vi "Main_PXI_v2.0.vi"() -> ()   [LabVIEW 2018]
doc: "Main VI for the controls"
uses:
  components/pmcl dynamic signal analyzer/Controls/DSA excitation specs.ctl
  components/pmcl dynamic signal analyzer/Controls/DSA cycle specs.ctl
  Typedefs/StateDef_Enum.ctl
  <vilib>/Utility/error.llb/DialogType.ctl
  <vilib>/Platform/TimedLoop/XDataNode/timing_clust.ctl
  <vilib>/Platform/TimedLoop/XDataNode/nitl_modes.ctl
  <vilib>/Platform/TimedLoop/XDataNode/wakeup.ctl
  <vilib>/DAQmx/read.llb/DAQmx Read (Analog 1D DBL NChan 1Samp).vi
  <vilib>/DAQmx/write.llb/DAQmx Write (Analog DBL 1Chan 1Samp).vi
  <vilib>/DAQmx/create/channels.llb/DAQmx Create Channel (AO-Voltage-Basic).vi
  <vilib>/DAQmx/create/channels.llb/DAQmx Create Channel (AI-Voltage-Basic).vi
  <vilib>/DAQmx/configure/timing.llb/DAQmx Timing (Sample Clock).vi
  <vilib>/DAQmx/create/timing.llb/DAQmx Create Timing Source (Control Loop From Task).vi
  <vilib>/DAQmx/miscellaneous.llb/DAQmx Fill In Error Info.vi
  <vilib>/Platform/TimedLoop/XDataNode/XDataNode.xnode
  Components/Timing/Timing.lvlib
  <vilib>/Platform/TimedLoop/XDataNode/XDNodeRunTimeDep.lvlib
  <vilib>/Analysis/NI_AALPro.lvlib
  <vilib>/ptbypt/NI_PtbyPt.lvlib
  <resource>/objmgr/daqmx.rc
  Components/Controller/Controller.lvlib
panel:
  in  "System Stop Button":bool
  in  "Pause chart?":bool
  in  "Controller Params":enum32{"Page 1"}(tab)
  in  "Kp":dbl=1.0 min=0.0
  in  "Controller On?":bool
  out "Status":string
  in  "Ref. Gen.":enum32{"Analog In", "Manual", "Wave Gen", "DSA"}(tab)=enum."Manual"
  in  "Ref. cmd.":dbl(slide) step=1.0 scale=-10.0..10.0 scale format="%#.1f"
  in  "Signal Cluster":T1={"phase"=0.0, "amplitude"=1.0, "frequency"=1.0, "offset"=1.0, "Signal"=enum."Square"} {"offset" format="%0.2f"; "frequency" format="%0.2f"; "amplitude" format="%0.2f"; "phase" format="%0.2f"}
  in  "Frequency\nResponse":enum16{"Plant", "RR", "CL"}(ring)
  out "DSA \nRunning?":bool
  in  "Stop \nDSA":bool
  in  "Start \nDSA":bool
  in  "DSA excitation specs":T2={"Initial Freq. [Hz]"=10.0, "Final Freq. [Hz]"=999.0, "# pts. in interval"=50, "Samping Time [s]"=0.001, "Amplitude [V]"=1.0, "Offset [V]"=0.0, "Freq Units (F: rad/s, T: Hz)"=TRUE}
  in  "Cycle Specs":T3={"Cycles To \nSettle (M)"=5, "Cycles To \nCalculate (N)"=10}
  in  "Loop Timing":enum32{"Ctrl.", "Ref. gen", "UI"}(tab)
  in  "ConvLateErrToWarning?":bool=TRUE
  in  "Ctrl.\nLoop Rate (Hz)":dbl=25000.0 format="%#_4p"
  out "# Finished\nLate counter":dbl
  out "# Finished\nLate counter":dbl
  in  "Ref. Gen.\nLoop Rate (Hz)":dbl=20000.0 format="%#_4p"
  in  "UI Loop rate (Hz)":dbl=1000.0 format="%#_6p"
  in  "Display Waveforms":enum32{"Controller Signals", "DSA "}(tab)
  out "Control Effort":dbl(graph)
  out "Waveform Chart":cluster{"Double":dbl, "Numeric":dbl}(graph)
  out "Phase Bode Plot":cluster{dbl[], dbl[]}(graph)
  out "Magnitude Bode Plot":cluster{dbl[], dbl[]}(graph)
  out "DSA Signals":cluster{"Double":dbl, "Double":dbl}(graph)
  # "Connect the Reference Signal \nto C/AI 1 of the myRIO."
  # "Pinout Config.:\nPort C/AI0 : Plant output being read           by the controller.\nPort C/AI1 : Reference signal for the control loop.\nPort C/AO0 : Control effort signal to the plant."
  # "Control Loop Timing"
  # "Ref.  Gen. Loop Timing"
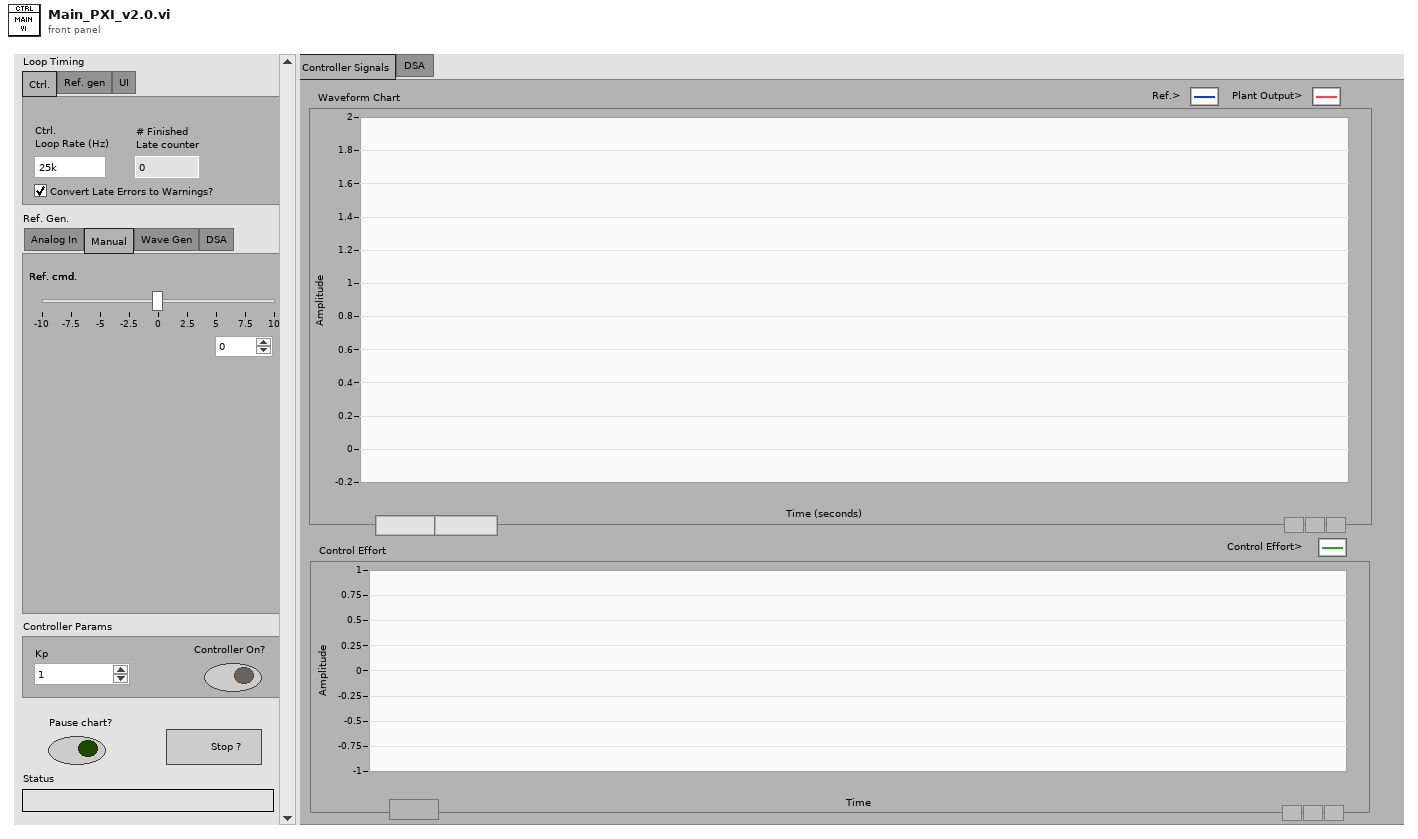
[diagram p1: front panel]
types:
  T1 = cluster{"phase":dbl, "amplitude":dbl, "frequency":dbl, "offset":dbl, "Signal":enum16{"Sine", "Square", "Sawtooth"}}
  T2 = typedef "DSA excitation specs.ctl" = cluster{"Initial Freq. [Hz]":dbl, "Final Freq. [Hz]":dbl, "# pts. in interval":i16, "Samping Time [s]":dbl, "Amplitude [V]":dbl, "Offset [V]":dbl, "Freq Units (F: rad/s, T: Hz)":bool}
  T3 = typedef "DSA cycle specs.ctl" = cluster{"Cycles To \nSettle (M)":i16, "Cycles To \nCalculate (N)":i16}
  T4 = typedef "DialogType.ctl" = u16
  T5 = typedef "StateDef_Enum.ctl" = enum16{"Initialize", "Wait", "Shutdown"}
  T6 = typedef "XDNodeRunTimeDep.lvlib/timing_clust.ctl" = cluster{"Expected End [f-1]":u64, "Actual End [f-1]":u64, "Finished Late? [f-1]":bool, "Expected End [i-1]":u64, "Actual End [i-1]":u64, "Finished Late? [i-1]":bool, "Expected Start [i]":u64, "Actual Start [i]":u64, "Expected Start [f]":u64, "Actual Start [f]":u64, "Source Name":string, "Structure Name":string, "Period":i64, "Deadline":i64, "Offset":i64, "Start":i64, "Priority":i32, "Timeout":i32, "Mode":T7, "Wakeup Reason":T8, "Error":errorcluster, "Source Type":string, "Secondary Source Type":string, "Global End Time":u64, "Global Start Time":u64, "Frame Duration":u64, "Iteration Duration":u64, "Assigned CPU":i32, "I/O Scan Engine Mode":u32}
  T7 = typedef "XDNodeRunTimeDep.lvlib/nitl_modes.ctl" = enum32{"No Change", "Process missed periods, maintain original phase", "Discard missed periods, maintain original phase", "Process missed periods, ignore original phase", "Discard missed periods, ignore original phase"}
  T8 = typedef "XDNodeRunTimeDep.lvlib/wakeup.ctl" = enum32{"Normal", "Aborted", "Asynchronous wakeup", "Timing source error", "Timed loop error", "Timeout"}
  T9 = cluster{"Analog In CH1":dbl, "Analog In CH0":dbl}
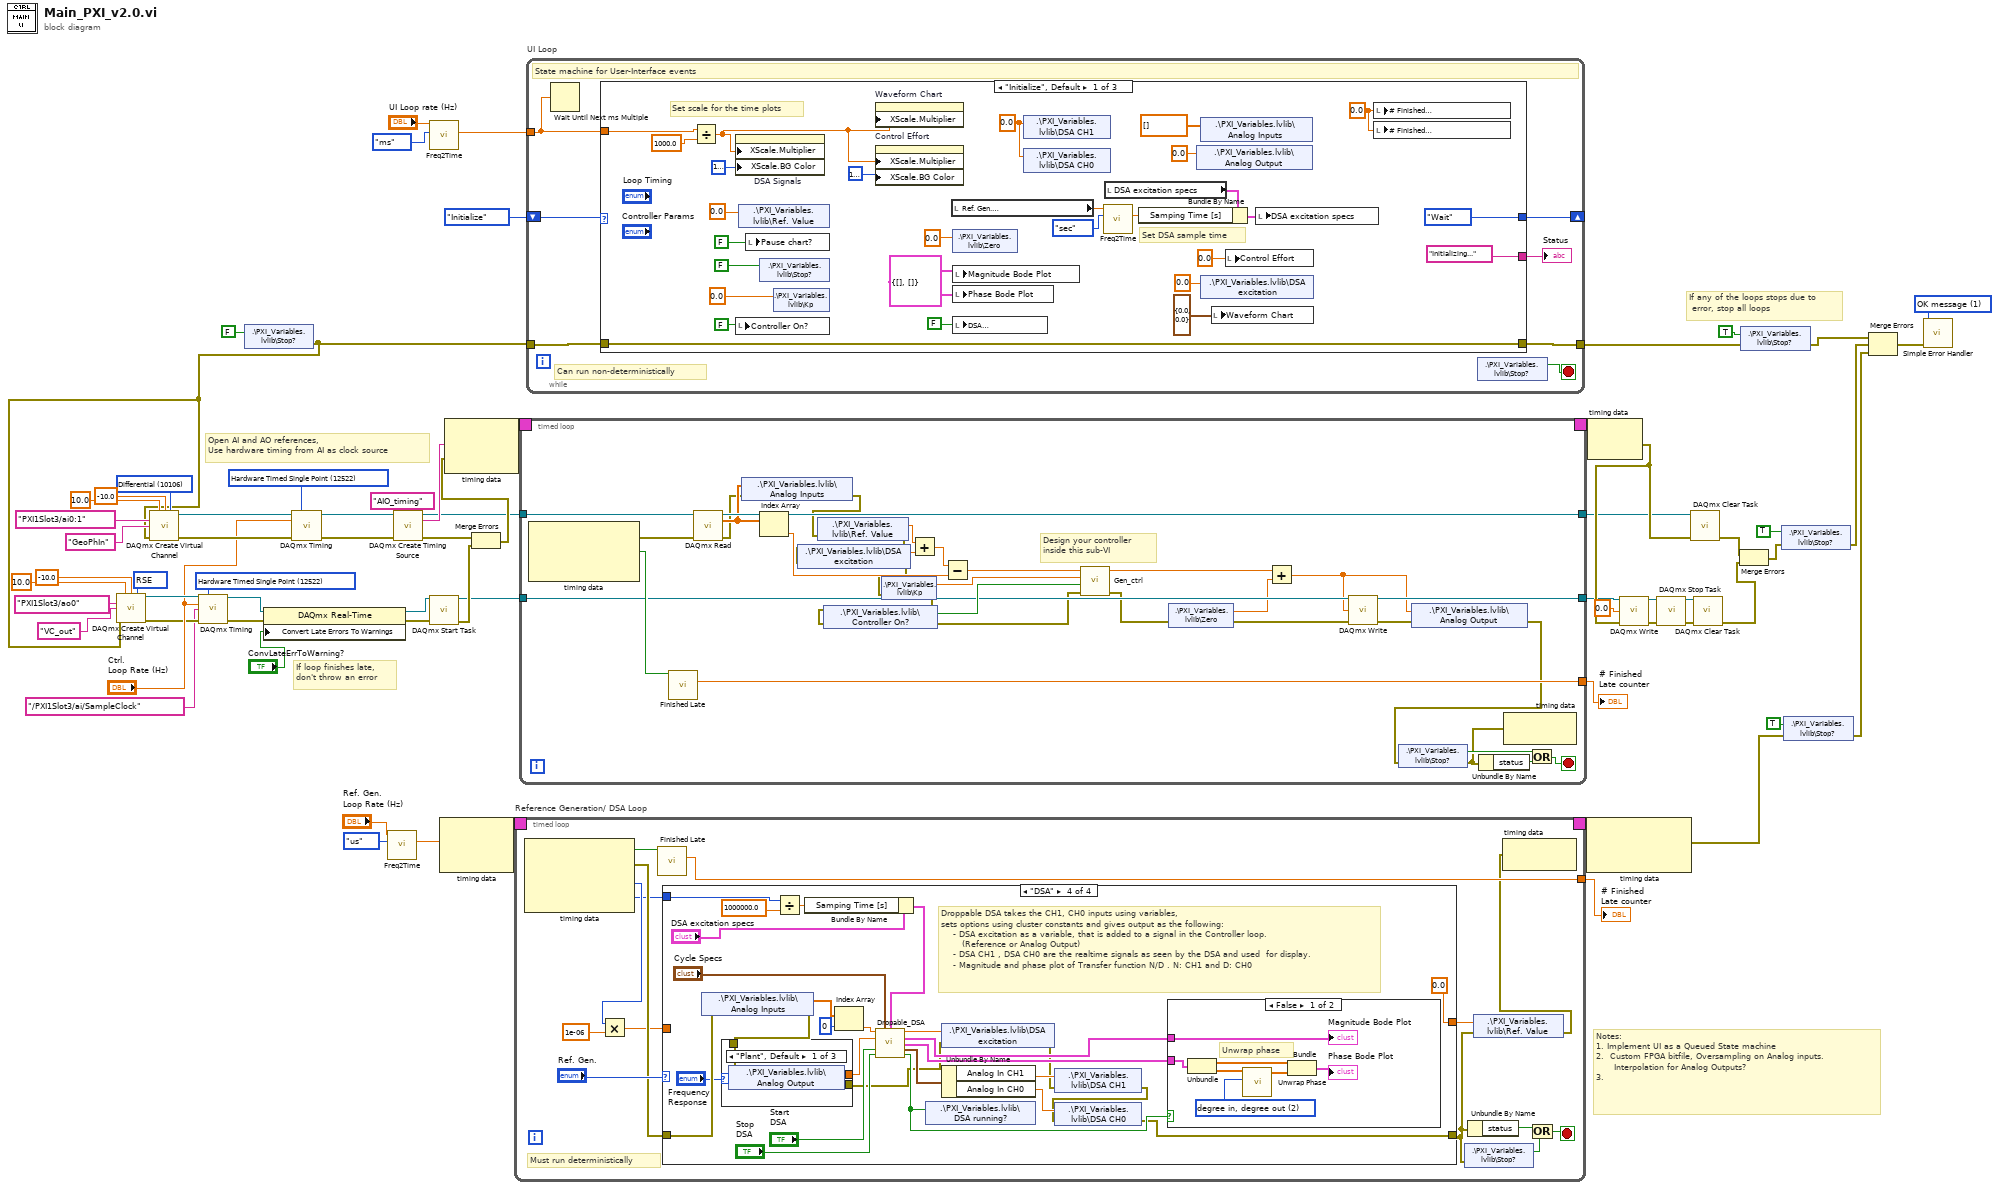
[diagram p0: block diagram]
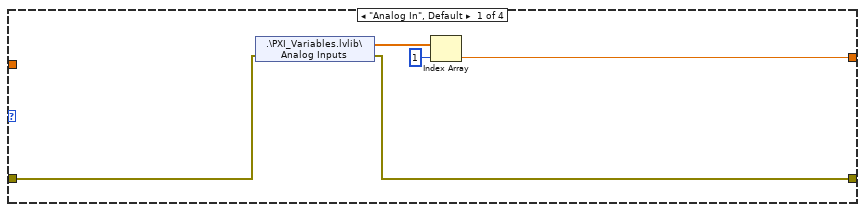
[diagram p2: hidden frame]
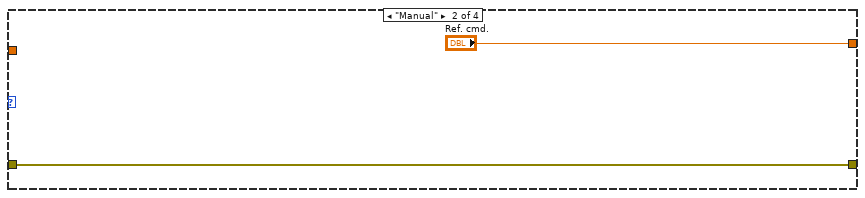
[diagram p3: hidden frame]
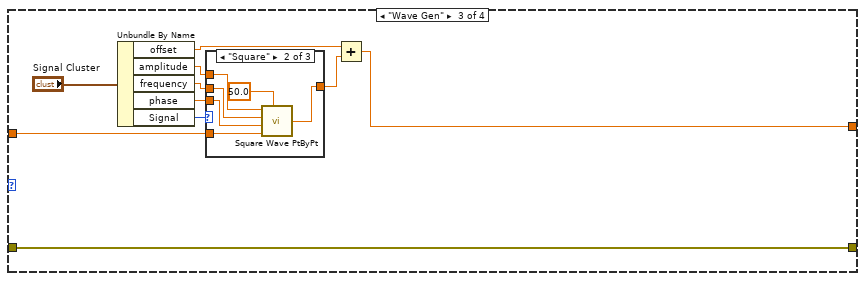
[diagram p4: hidden frame]
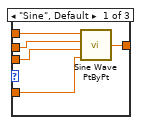
[diagram p5: hidden frame]
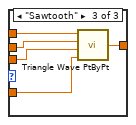
[diagram p6: hidden frame]
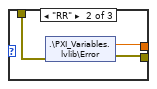
[diagram p7: hidden frame]
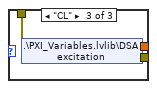
[diagram p8: hidden frame]
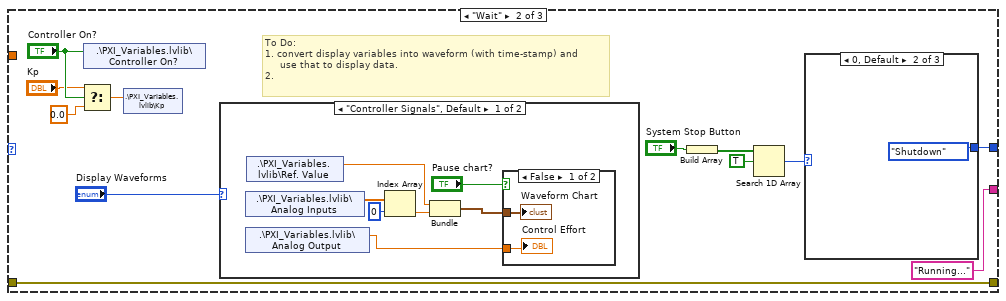
[diagram p10: hidden frame]
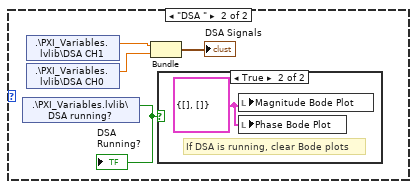
[diagram p12: hidden frame]
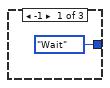
[diagram p14: hidden frame]
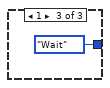
[diagram p15: hidden frame]
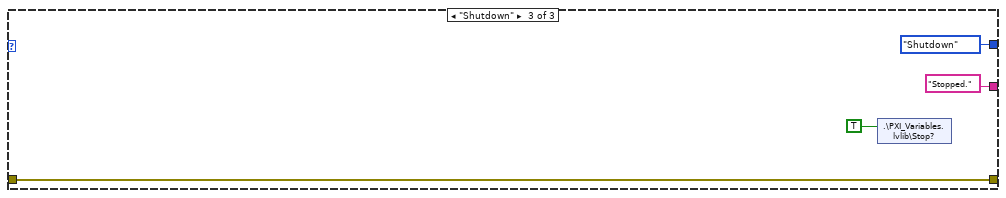
[diagram p16: hidden frame]
diagram:
  w7 = 12522 items=["Finite Samples"=10178, "Continuous Samples"=10123, "Hardware Timed Single Point"=12522] ("sample mode")
  w13 = T4 1 items=["no dialog", "OK message", "continue or stop message", "OK message + warnings", "continue/stop + warnings"] ("type of dialog (OK msg:1)")
  w22 = 12522 items=["Finite Samples"=10178, "Continuous Samples"=10123, "Hardware Timed Single Point"=12522] ("sample mode")
  w47 = 10106 items=["Default"=-1, "RSE"=10083, "NRSE"=10078, "Differential"=10106, "Pseudodifferential"=12529] ("input terminal configuration")
  w51 = 10083 items=["Default"=-1, "RSE"=10083, "Differential"=10106, "Pseudodifferential"=12529] ("output terminal configuration")
  # "If loop finishes late,\ndon't throw an error"
  # "Open AI and AO references,\nUse hardware timing from AI as clock source"
  # "Notes:\n1. Implement UI as a Queued State machine\n2.  Custom FPGA bitfile, Oversampling on Analog inputs. \n      Interpolation for Analog Outputs?\n3."
  # "If any of the loops stops due to\n error, stop all loops"
  n1 = shared-variable ".\\PXI_Variables.lvlib\\Stop?"(FALSE ("Stop?")) -> (error out=w4:errorcluster)  [unwired: 1 in]
  n2 = call-poly <vilib>:"DAQmx Create Virtual Channel.vi"("maximum value"=10.0, "minimum value"=-10.0, "output terminal configuration"=w51, "physical channels"=tag "PXI1Slot3/ao0", "name to assign"="VC_out", "error in"=w4) -> ("task out"=w12:refnum<k21>, "error out"=w8:errorcluster)  [unwired: 8 in]
  n3 = call-poly <vilib>:"DAQmx Create Virtual Channel.vi"("maximum value"=10.0, "minimum value"=-10.0, "input terminal configuration"=w47, "physical channels"=tag "PXI1Slot3/ai0:1", "name to assign"="GeoPhIn", "error in"=w4) -> ("task out"=w24:refnum<k21>, "error out"=w23:errorcluster)  [unwired: 8 in]
  n4 = call-poly <vilib>:"DAQmx Timing.vi"("task/channels in"=w12, "sample mode"=w7, "rate"="Ctrl.\nLoop Rate (Hz)", "source"=tag "/PXI1Slot3/ai/SampleClock", "error in"=w8) -> ("task out"=w10:refnum<k21>, "error out"=w9:errorcluster)  [unwired: 9 in]
  n5 = property class="DAQmx Real-Time"(reference=w10, error in=w9, "Convert Late Errors To Warnings"="ConvLateErrToWarning?") -> (reference out=w15:refnum<k21>, error out=w20:errorcluster)
  n6 = call-poly <vilib>:"DAQmx Timing.vi"("task/channels in"=w24, "sample mode"=w22, "rate"="Ctrl.\nLoop Rate (Hz)", "error in"=w23) -> ("task out"=w14:refnum<k21>, "error out"=w17:errorcluster)  [unwired: 10 in]
  n7 = call "Freq2Time.vi"("Int. Time Unit"=enum16{"sec", "us", "ms"}."us", "Sample rate (Hz)"="Ref. Gen.\nLoop Rate (Hz)") -> ("Int.  time [unit]"=w3:dbl)  [unwired: 7 in, 2 out]
  n8 = call-poly <vilib>:"DAQmx Create Timing Source.vi"("task/channels in"=w14, "timing source name"="AIO_timing", "error in"=w17) -> ("task out"=w18:refnum<k21>, "timing source out"=w19:string, "error out"=w16:errorcluster)  [unwired: 10 in]
  n9 = call "Freq2Time.vi"("Int. Time Unit"=enum16{"sec", "us", "ms"}."ms", "Sample rate (Hz)"="UI Loop rate (Hz)") -> ("Int.  time [unit]"=w59:dbl)  [unwired: 7 in, 2 out]
  n10 = call <vilib>:"DAQmx Start Task.vi"("task/channels in"=w15, "error in"=w20) -> ("task out"=w26:refnum<k21>, "error out"=w49:errorcluster)  [unwired: 12 in]
  n11 = node-c288(w3) -> (w66:T6)  [unwired: 1 in]
  n12 = Merge Errors(w16, w49) -> (w41:errorcluster)
  n13 = node-c288(w19, w41) -> (w43:T6)
  n14 = timed-loop "Reference Generation/ DSA Loop" {
    timing: w66 -> [_]
    timing-out: [_] -> w65
    tunnel: [w81] -> w64
    stop <- w75 stop-if-true
    # "Must run deterministically"
    n15 = node-c288() -> (w82:bool, w78:errorcluster, w72:i64, w71:i64)  [unwired: 1 in]
    n16 = Multiply(x=w72, y=1e-06) -> (x*y=w74:dbl)
    n17 = call "Finished Late.vi"("Finished \nLate?"=w82) -> ("# Finished\nLate counter"=w81:dbl)  [unwired: 8 in, 2 out]
    n18 = case shown="\"DSA\"" "Ref. Gen." {
      tunnel: [w87 "Ref. cmd." w92 0.0 ("Ref. cmd.")] -> w79
      tunnel: w78 -> [w85 w88 w91 w122]
      tunnel: [w84 w88 w91 w125] -> w69
      tunnel: w74 -> [_ _ w90 _]
      tunnel: w71 -> [_ _ _ w132]
      frame "Analog In", Default {
        n19 = shared-variable ".\\PXI_Variables.lvlib\\Analog Inputs"(error in=w85) -> (w86:dbl[], error out=w84:errorcluster)
        n20 = Index Array(array=w86, index=1) -> (element=w87:dbl)
      }
      frame "Manual" {
      }
      frame "Wave Gen" {
        n21 = Unbundle By Name("Signal Cluster") -> ("offset"=w93:dbl, "amplitude"=w96:dbl, "frequency"=w95:dbl, "phase"=w94:dbl, "Signal"=w97:enum16{"Sine", "Square", "Sawtooth"})
        n22 = case shown="\"Square\"" w97 {
          tunnel: [w104 w109 w115] -> w99
          tunnel: w96 -> [w103 w108 w114]
          tunnel: w95 -> [w102 w107 w113]
          tunnel: w94 -> [w101 w106 w112]
          tunnel: w90 -> [w100 w105 w111]
          frame "Sine", Default {
            n23 = call <vilib>:"Sine Wave PtByPt.vi"("time"=w100, "phase"=w101, "frequency"=w102, "amplitude"=w103) -> ("sine wave"=w104:dbl)
          }
          frame "Square" {
            n24 = call <vilib>:"Square Wave PtByPt.vi"("amplitude"=w108, "frequency"=w107, "phase"=w106, "time"=w105, "duty cycle (%)"=50.0) -> ("square wave"=w109:dbl)
          }
          frame "Sawtooth" {
            n25 = call <vilib>:"Triangle Wave PtByPt.vi"("time"=w111, "phase"=w112, "frequency"=w113, "amplitude"=w114) -> ("triangle wave"=w115:dbl)
          }
        }
        n26 = Add(x=w93, y=w99) -> (x+y=w92:dbl)
      }
      frame "DSA" {
        # "Droppable DSA takes the CH1, CH0 inputs using variables, \nsets options using cluster constants and gives output as the following:\n    - DSA excitation as a variable, that is added to a signal in the Controller loop. \n       (Reference or Analog Output)\n    - DSA CH1 , DSA CH0 are the realtime signals as seen by the DSA and used  for display.\n    - Magnitude and phase plot of Transfer function N/D . N: CH1 and D: CH0"
        n27 = shared-variable ".\\PXI_Variables.lvlib\\Analog Inputs"(error in=w122) -> (w121:dbl[], error out=w119:errorcluster)
        n28 = case shown="\"Plant\", Default" "Frequency\nResponse" {
          tunnel: [w145 w148 w149] -> w120
          tunnel: w119 -> [w144 w146 w151]
          tunnel: [w143 w147 w150] -> w116
          frame "Plant", Default {
            n29 = shared-variable ".\\PXI_Variables.lvlib\\Analog Output"(error in=w144) -> (w145:dbl, error out=w143:errorcluster)
          }
          frame "RR" {
            n30 = shared-variable ".\\PXI_Variables.lvlib\\Error"(error in=w146) -> (w148:dbl, error out=w147:errorcluster)
          }
          frame "CL" {
            n31 = shared-variable ".\\PXI_Variables.lvlib\\DSA excitation"(error in=w151) -> (w149:dbl, error out=w150:errorcluster)
          }
        }
        n32 = Divide(x=w132, y=1000000.0) -> (x/y=w130:dbl)
        n33 = Bundle By Name(cluster="DSA excitation specs", "Samping Time [s]"=w130) -> (w129:T2)
        n34 = Index Array(array=w121, index=0) -> (element=w123:dbl)
        n35 = call "Dropable_DSA.vi"("Analog In CH1"=w123, "Cycle Specs"="Cycle Specs", "Excitation Specs"=w129, "Analog In CH0"=w120, "START"="Start \nDSA", "STOP"="Stop \nDSA") -> ("Analog Out"=w141:dbl, "Bode Magnitude"=w134:cluster{dbl[], dbl[]}, "Bode Phase"=w133:cluster{dbl[], dbl[]}, "Live signals"=w138:T9, "Running"=w128:bool)  [unwired: 4 in, 1 out]
        n36 = shared-variable ".\\PXI_Variables.lvlib\\DSA running?"(w128) -> ()  [unwired: 1 in, 1 out]
        n37 = shared-variable ".\\PXI_Variables.lvlib\\DSA excitation"(w141, error in=w116) -> (error out=w127:errorcluster)
        n38 = Unbundle By Name(w138) -> ("Analog In CH1"=w137:dbl, "Analog In CH0"=w136:dbl)
        n39 = shared-variable ".\\PXI_Variables.lvlib\\DSA CH1"(w137, error in=w127) -> (error out=w126:errorcluster)
        n40 = shared-variable ".\\PXI_Variables.lvlib\\DSA CH0"(w136, error in=w126) -> (error out=w125:errorcluster)
        n41 = case shown="False" w128 {
          tunnel: w134 -> [w152 _]
          tunnel: w133 -> [w154 _]
          frame False {
            w156 = 2 items=["radian in, radian out", "radian in, degree out", "degree in, degree out", "degree in, radian out"] ("phase unit")
            # "Unwrap phase"
            n42 = Unbundle(w154) -> (w158:dbl[], w155:dbl[])
            n43 = call <vilib>:"Unwrap Phase.vi"("phase unit"=w156, "Phase"=w155) -> ("Unwrapped Phase"=w157:dbl[])  [unwired: 8 in, 1 out]
            n44 = Bundle(w158, "Unwrapped Phase"=w157) -> (→"Phase Bode Plot":cluster{dbl[], "Unwrapped Phase":dbl[]})  [unwired: 1 in]
            "Magnitude Bode Plot" <- w152
          }
          frame True {
          }
        }
      }
    }
    n45 = shared-variable ".\\PXI_Variables.lvlib\\Stop?"(error in=w69) -> (w76:bool)  [unwired: 1 out]
    n46 = Unbundle By Name(w69) -> ("status"=w77:bool)
    n47 = shared-variable ".\\PXI_Variables.lvlib\\Ref. Value"(w79, error in=w69) -> (error out=w70:errorcluster)
    n48 = node-c288(w70) -> ()  [unwired: 1 out]
    n49 = Or(x=w77, y=w76) -> (x .or. y?=w75:bool)
  }
  "# Finished\nLate counter" <- w64
  n50 = timed-loop {
    timing: w43 -> [_]
    timing-out: [_] -> w42
    tunnel: w18 -> [w197]
    tunnel: [w195] -> w28
    tunnel: [w194] -> w27
    tunnel: w26 -> [w181]
    tunnel: [w180] -> w25
    stop <- w182 stop-if-true
    # "Design your controller \ninside this sub-VI"
    n51 = node-c288() -> (w198:errorcluster, w196:bool)  [unwired: 1 in, 1 out]
    n52 = call "Finished Late.vi"("Finished \nLate?"=w196) -> ("# Finished\nLate counter"=w195:dbl)  [unwired: 8 in, 2 out]
    n53 = call-poly <vilib>:"DAQmx Read.vi"("task/channels in"=w197, "error in"=w198) -> ("task out"=w194:refnum<k21>, "data"=w193:dbl[], "error out"=w178:errorcluster)  [unwired: 11 in]
    n54 = shared-variable ".\\PXI_Variables.lvlib\\Analog Inputs"(w193, error in=w178) -> (error out=w177:errorcluster)
    n55 = Index Array(array=w193) -> (element=w192:dbl)  [unwired: 1 in]
    n56 = shared-variable ".\\PXI_Variables.lvlib\\Ref. Value"(error in=w177) -> (w190:dbl, error out=w176:errorcluster)
    n57 = shared-variable ".\\PXI_Variables.lvlib\\DSA excitation"(error in=w176) -> (w189:dbl, error out=w175:errorcluster)
    n58 = shared-variable ".\\PXI_Variables.lvlib\\Kp"(error in=w175) -> (w187:dbl, error out=w174:errorcluster)
    n59 = shared-variable ".\\PXI_Variables.lvlib\\Controller On?"(error in=w174) -> (w186:bool, error out=w173:errorcluster)
    n60 = Add(x=w190, y=w189) -> (x+y=w191:dbl)
    n61 = Subtract(x=w191, y=w192) -> (x-y=w188:dbl)
    n62 = call "Gen_ctrl.vi"("error in (no error)"=w173, "Controller On?"=w186, "Kp"=w187, "Error In"=w188) -> ("error out"=w172:errorcluster, "Ctrl Effort Out"=w170:dbl)  [unwired: 6 in]
    n63 = shared-variable ".\\PXI_Variables.lvlib\\Zero"(error in=w172) -> (w169:dbl, error out=w171:errorcluster)
    n64 = Add(x=w170, y=w169) -> (x+y=w179:dbl)
    n65 = call-poly <vilib>:"DAQmx Write.vi"("task/channels in"=w181, "data"=w179, "error in"=w171) -> ("task out"=w180:refnum<k21>, "error out"=w168:errorcluster)  [unwired: 10 in, 1 out]
    n66 = shared-variable ".\\PXI_Variables.lvlib\\Analog Output"(w179, error in=w168) -> (error out=w167:errorcluster)
    n67 = shared-variable ".\\PXI_Variables.lvlib\\Stop?"(error in=w167) -> (w185:bool, error out=w184:errorcluster)
    n68 = Unbundle By Name(w184) -> ("status"=w183:bool)
    n69 = node-c288(w184) -> ()  [unwired: 1 out]
    n70 = Or(x=w185, y=w183) -> (x .or. y?=w182:bool)
  }
  "# Finished\nLate counter" <- w28
  n71 = while "UI Loop" {
    shift-right: [w210] -> _
    shift-left: StateDef_Enum."Initialize" ("State defining Enum") -> [w211]
    tunnel: w4 -> [w209]
    tunnel: [w208] -> w58
    tunnel: w59 -> [w205]
    stop <- w206 stop-if-true
    # "Can run non-deterministically"
    # "State machine for User-Interface events"
    n72 = Wait Until Next ms Multiple(millisecond multiple=w205) -> ()  [unwired: 1 out]
    n73 = case shown="\"Initialize\", Default" w211 {
      tunnel: [StateDef_Enum."Wait" ("State defining Enum") w248 StateDef_Enum."Shutdown" ("State defining Enum")] -> w210
      tunnel: w209 -> [w236 w246 w272]
      tunnel: [w236 w246 w272] -> w208
      tunnel: ["Initializing..." ("Status") "Running..." ("Status") "Stopped." ("Status")] -> w207
      tunnel: w205 -> [w234 _ _]
      frame "Initialize", Default {
        w212 = 0.0 ("# Finished\nLate counter")
        w213 = 0.0 ("DSA CH1")
        w229 = cluster{dbl[], dbl[]} {[], []} ("Magnitude Bode Plot")
        # "Set DSA sample time"
        # "Set scale for the time plots"
        n74 = Divide(x=w234, y=1000.0) -> (x/y=w221:dbl)
        n75 = property on="DSA Signals" class="WFChart (strict)"("XScale.Multiplier"=w221, "XScale.BG Color"=u32 16777216) -> ()  [unwired: 2 in, 2 out]
        n76 = local write "Controller On?"(FALSE ("Controller On?")) -> ()
        n77 = shared-variable ".\\PXI_Variables.lvlib\\Ref. Value"(0.0 ("Ref. Value")) -> ()  [unwired: 1 in, 1 out]
        n78 = local write "Pause chart?"(FALSE ("Pause chart?")) -> ()
        n79 = shared-variable ".\\PXI_Variables.lvlib\\Stop?"(FALSE ("Stop?")) -> ()  [unwired: 1 in, 1 out]
        n80 = shared-variable ".\\PXI_Variables.lvlib\\Kp"(0.0 ("Kp")) -> ()  [unwired: 1 in, 1 out]
        n81 = property on="Waveform Chart" class="WFChart (strict)"("XScale.Multiplier"=w221) -> ()  [unwired: 2 in, 2 out]
        n82 = property on="Control Effort" class="WFChart (strict)"("XScale.Multiplier"=w221, "XScale.BG Color"=u32 16777216) -> ()  [unwired: 2 in, 2 out]
        n83 = local read "Ref. Gen.\nLoop Rate (Hz)"() -> (w224:dbl)
        n84 = shared-variable ".\\PXI_Variables.lvlib\\Zero"(0.0 ("Zero")) -> ()  [unwired: 1 in, 1 out]
        n85 = local write "Magnitude Bode Plot"(w229) -> ()
        n86 = local write "Phase Bode Plot"(w229) -> ()
        n87 = local write "DSA \nRunning?"(FALSE ("DSA \nRunning?")) -> ()
        n88 = shared-variable ".\\PXI_Variables.lvlib\\DSA CH1"(w213) -> ()  [unwired: 1 in, 1 out]
        n89 = shared-variable ".\\PXI_Variables.lvlib\\DSA CH0"(w213) -> ()  [unwired: 1 in, 1 out]
        n90 = call "Freq2Time.vi"("Int. Time Unit"=enum16{"sec", "us", "ms"}."sec", "Sample rate (Hz)"=w224) -> ("Int.  time [unit]"=w222:dbl)  [unwired: 7 in, 2 out]
        n91 = local read "DSA excitation specs"() -> (w226:T2)
        n92 = Bundle By Name(cluster=w226, "Samping Time [s]"=w222) -> (w225:T2)
        n93 = shared-variable ".\\PXI_Variables.lvlib\\Analog Output"(0.0 ("Analog Output")) -> ()  [unwired: 1 in, 1 out]
        n94 = shared-variable ".\\PXI_Variables.lvlib\\Analog Inputs"(dbl[] [] ("Analog Inputs")) -> ()  [unwired: 1 in, 1 out]
        n95 = shared-variable ".\\PXI_Variables.lvlib\\DSA excitation"(0.0 ("DSA excitation")) -> ()  [unwired: 1 in, 1 out]
        n96 = local write "Waveform Chart"(cluster{"Double":dbl, "Numeric":dbl} {"Double"=0.0, "Numeric"=0.0} ("Waveform Chart")) -> ()
        n97 = local write "Control Effort"(0.0 ("Control Effort")) -> ()
        n98 = local write "DSA excitation specs"(w225) -> ()
        n99 = local write "# Finished\nLate counter"(w212) -> ()
        n100 = local write "# Finished\nLate counter"(w212) -> ()
      }
      frame "Wait" {
        # "To Do:\n1. convert display variables into waveform (with time-stamp) and\n     use that to display data.\n2."
        n101 = Select(t="Kp", s="Controller On?", f=0.0) -> (s? t:f=w244:dbl)
        n102 = shared-variable ".\\PXI_Variables.lvlib\\Controller On?"("Controller On?") -> ()  [unwired: 1 in, 1 out]
        n103 = shared-variable ".\\PXI_Variables.lvlib\\Kp"(w244) -> ()  [unwired: 1 in, 1 out]
        n104 = case shown="\"Controller Signals\", Default" "Display Waveforms" {
          frame "Controller Signals", Default {
            n105 = shared-variable ".\\PXI_Variables.lvlib\\Analog Inputs"() -> (w258:dbl[])  [unwired: 1 in, 1 out]
            n106 = shared-variable ".\\PXI_Variables.lvlib\\Analog Output"() -> (w252:dbl)  [unwired: 1 in, 1 out]
            n107 = shared-variable ".\\PXI_Variables.lvlib\\Ref. Value"() -> (w255:dbl)  [unwired: 1 in, 1 out]
            n108 = Index Array(array=w258, index=0) -> (element=w257:dbl)
            n109 = Bundle("Double"=w255, "Numeric"=w257) -> (w253:cluster{"Double":dbl, "Numeric":dbl})  [unwired: 1 in]
            n110 = case shown="False" "Pause chart?" {
              tunnel: w253 -> [w260 _]
              tunnel: w252 -> [w259 _]
              frame False {
                "Waveform Chart" <- w260
                "Control Effort" <- w259
              }
              frame True {
              }
            }
          }
          frame "DSA " {
            n111 = shared-variable ".\\PXI_Variables.lvlib\\DSA running?"() -> (w261:bool)  [unwired: 1 in, 1 out]
            "DSA \nRunning?" <- w261
            n112 = shared-variable ".\\PXI_Variables.lvlib\\DSA CH1"() -> (w263:dbl)  [unwired: 1 in, 1 out]
            n113 = shared-variable ".\\PXI_Variables.lvlib\\DSA CH0"() -> (w262:dbl)  [unwired: 1 in, 1 out]
            n114 = Bundle("Double"=w263, "Double"=w262) -> (→"DSA Signals":cluster{"Double":dbl, "Double":dbl})  [unwired: 1 in]
            n115 = case shown="True" w261 {
              frame False {
              }
              frame True {
                w265 = cluster{dbl[], dbl[]} {[], []} ("Magnitude Bode Plot")
                # "If DSA is running, clear Bode plots"
                n116 = local write "Magnitude Bode Plot"(w265) -> ()
                n117 = local write "Phase Bode Plot"(w265) -> ()
              }
            }
          }
        }
        n118 = Build Array("System Stop Button") -> (w250:bool[])
        n119 = Search 1D Array(1D array=w250, element=TRUE) -> (index of element=w247:i32)  [unwired: 1 in]
        n120 = case shown="0, Default" w247 {
          tunnel: [StateDef_Enum."Wait" ("State defining Enum") StateDef_Enum."Shutdown" ("State defining Enum") StateDef_Enum."Wait" ("State defining Enum")] -> w248
          frame -1 {
          }
          frame 0, Default {
          }
          frame 1 {
          }
        }
      }
      frame "Shutdown" {
        n121 = shared-variable ".\\PXI_Variables.lvlib\\Stop?"(TRUE) -> ()  [unwired: 1 in, 1 out]
      }
    }
    "Status" <- w207
    n122 = shared-variable ".\\PXI_Variables.lvlib\\Stop?"() -> (w206:bool)  [unwired: 1 in, 1 out]
  }
  n123 = node-c288(w65) -> (w63:errorcluster)  [unwired: 1 out]
  n124 = node-c288(w42) -> (w31:errorcluster)
  n125 = call-poly <vilib>:"DAQmx Write.vi"("task/channels in"=w25, "data"=0.0, "error in"=w31) -> ("task out"=w37:refnum<k21>, "error out"=w36:errorcluster)  [unwired: 10 in, 1 out]
  n126 = call <vilib>:"DAQmx Stop Task.vi"("task/channels in"=w37, "error in"=w36) -> ("task out"=w35:refnum<k21>, "error out"=w34:errorcluster)  [unwired: 12 in]
  n127 = call <vilib>:"DAQmx Clear Task.vi"("task in"=w27, "error in"=w31) -> ("error out"=w32:errorcluster)  [unwired: 13 in]
  n128 = call <vilib>:"DAQmx Clear Task.vi"("task in"=w35, "error in"=w34) -> ("error out"=w33:errorcluster)  [unwired: 13 in]
  n129 = Merge Errors(w32, w33) -> (w39:errorcluster)
  n130 = shared-variable ".\\PXI_Variables.lvlib\\Stop?"(TRUE ("Stop?"), error in=w58) -> (error out=w57:errorcluster)
  n131 = shared-variable ".\\PXI_Variables.lvlib\\Stop?"(TRUE ("Stop?"), error in=w39) -> (error out=w29:errorcluster)
  n132 = shared-variable ".\\PXI_Variables.lvlib\\Stop?"(TRUE ("Stop?"), error in=w63) -> (error out=w30:errorcluster)
  n133 = Merge Errors(w57, w29, w30) -> (w67:errorcluster)
  n134 = call <vilib>:"Simple Error Handler.vi"("type of dialog (OK msg:1)"=w13, "error in (no error)"=w67) -> ()  [unwired: 3 in, 5 out]
